vi "R4DataCollection.vi"(8 "error constant":errorcluster, 10 "Write Once":bool, 11 "LabVIEW Web Service":refnum<class "Web Service.lvclass">) -> (0 "error out":errorcluster={"status"=FALSE, "code"=0, "source"="0"})   [LabVIEW 2016]
uses:
  <vilib>/wsapi/Web Service.lvclass
  <vilib>/Platform/TimedLoop/XDataNode/timing_clust.ctl
  <vilib>/Platform/TimedLoop/XDataNode/nitl_modes.ctl
  <vilib>/Platform/TimedLoop/XDataNode/wakeup.ctl
  <vilib>/Platform/TimedLoop/XDataNode/XDataNode.xnode
  <vilib>/Platform/TimedLoop/XDataNode/XDNodeRunTimeDep.lvlib
  <vilib>/ptbypt/NI_PtbyPt.lvlib
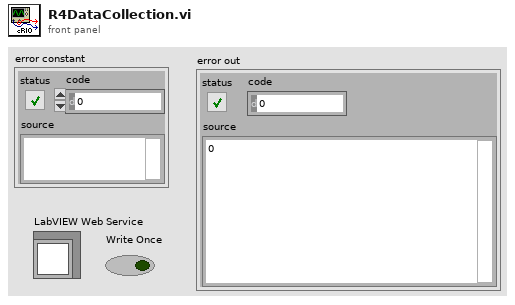
[diagram p1: front panel]
types:
  T1 = typedef "XDNodeRunTimeDep.lvlib/timing_clust.ctl" = cluster{"Expected End [f-1]":u64, "Actual End [f-1]":u64, "Finished Late? [f-1]":bool, "Expected End [i-1]":u64, "Actual End [i-1]":u64, "Finished Late? [i-1]":bool, "Expected Start [i]":u64, "Actual Start [i]":u64, "Expected Start [f]":u64, "Actual Start [f]":u64, "Source Name":string, "Structure Name":string, "Period":i64, "Deadline":i64, "Offset":i64, "Start":i64, "Priority":i32, "Timeout":i32, "Mode":T2, "Wakeup Reason":T3, "Error":errorcluster, "Source Type":string, "Secondary Source Type":string, "Global End Time":u64, "Global Start Time":u64, "Frame Duration":u64, "Iteration Duration":u64, "Assigned CPU":i32, "I/O Scan Engine Mode":u32}
  T2 = typedef "XDNodeRunTimeDep.lvlib/nitl_modes.ctl" = enum32{"No Change", "Process missed periods, maintain original phase", "Discard missed periods, maintain original phase", "Process missed periods, ignore original phase", "Discard missed periods, ignore original phase"}
  T3 = typedef "XDNodeRunTimeDep.lvlib/wakeup.ctl" = enum32{"Normal", "Aborted", "Asynchronous wakeup", "Timing source error", "Timed loop error", "Timeout"}
  T4 = cluster{"Media Pump":bool, "Water Pump":bool, "Gas Pump":bool, "Effluent Pump":bool, "Release Pump":bool}
  T5 = cluster{"Array of Double[0]":dbl, "Array of Double[1]":dbl, "Array of Double[2]":dbl, "Array of Double[3]":dbl, "Array of Double[4]":dbl, "Array of Double[5]":dbl, "Array of Double[6]":dbl, "Array of Double[7]":dbl, "Array of Double[8]":dbl}
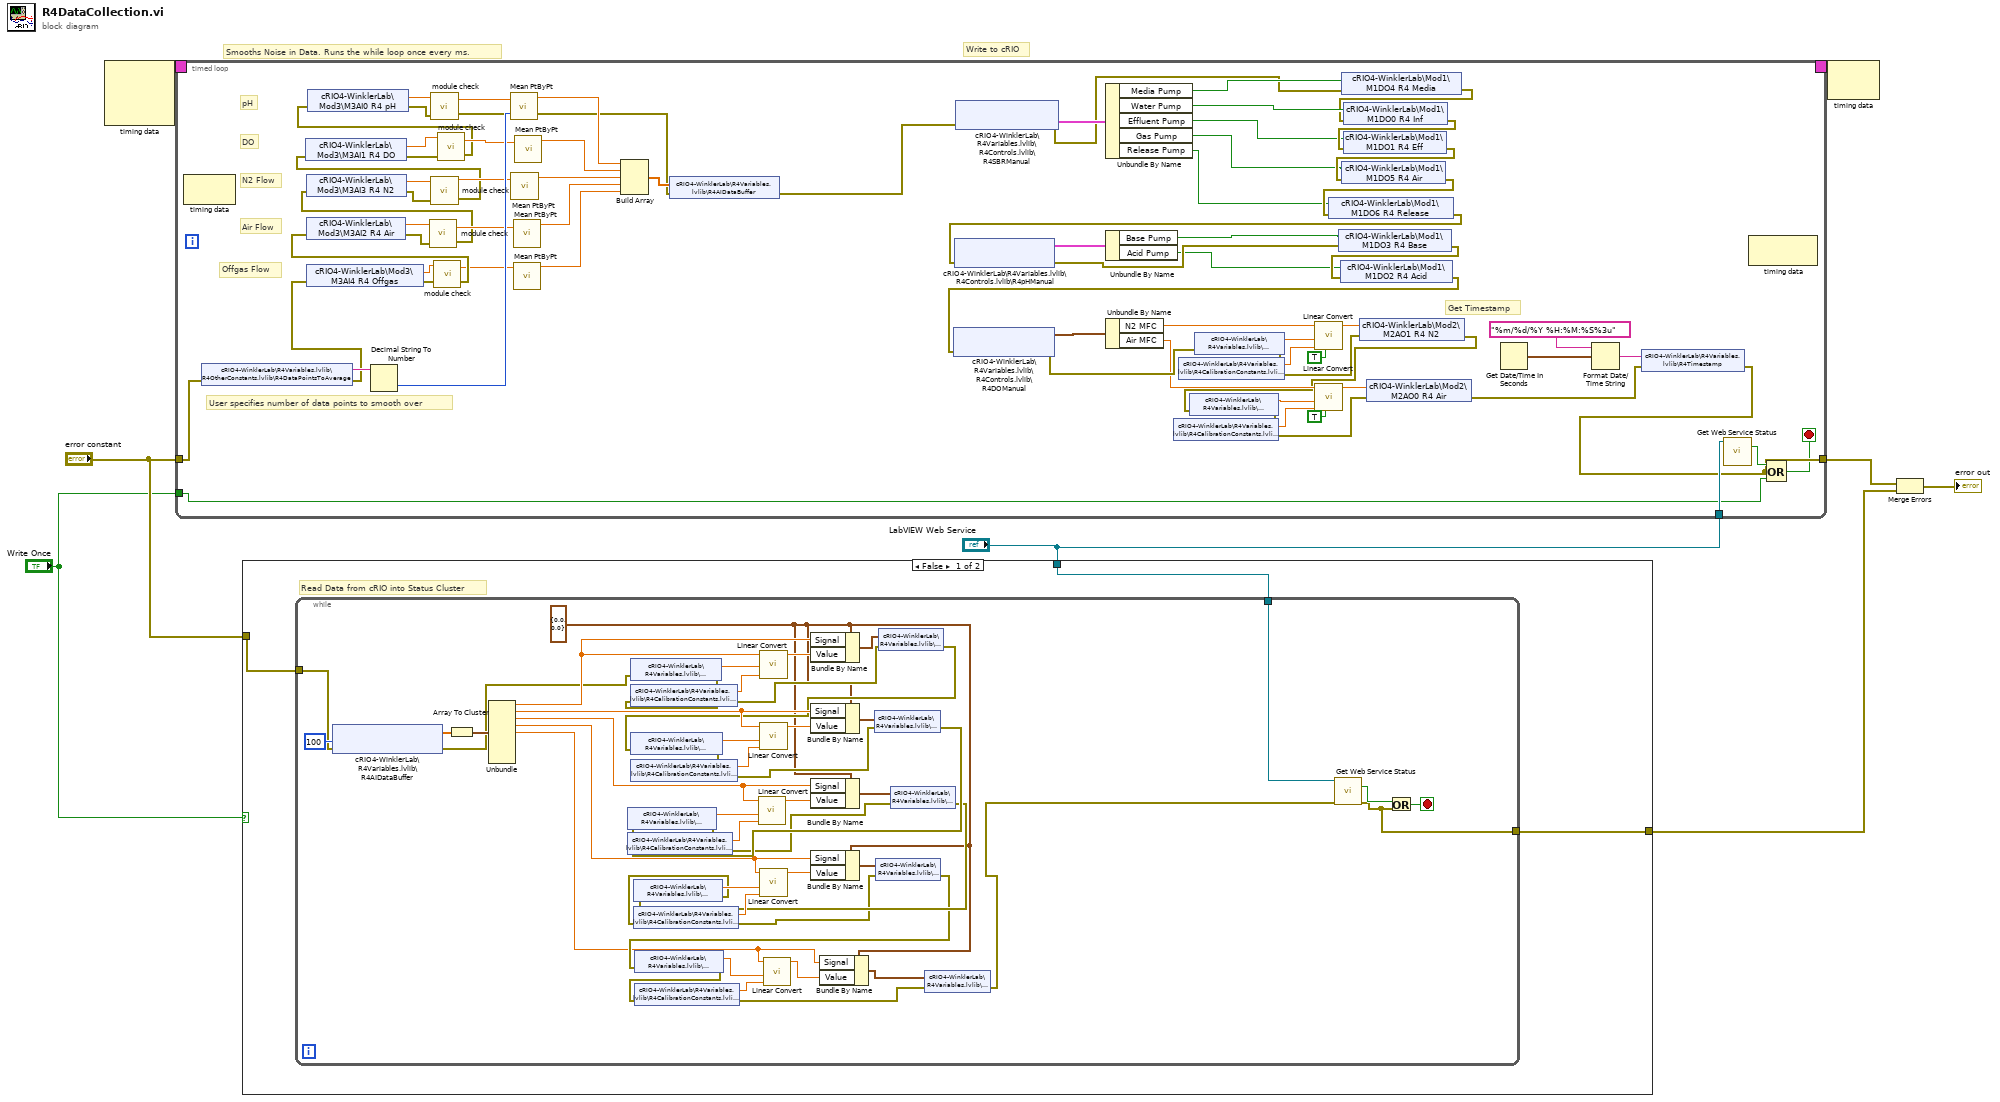
[diagram p0: block diagram]
diagram:
  # "Write to cRIO"
  # "Smooths Noise in Data. Runs the while loop once every ms."
  n1 = node-c288() -> (w8:T1)  [unwired: 3 in]
  n2 = timed-loop {
    timing: w8 -> [_]
    timing-out: [_] -> w7
    tunnel: "error constant" -> [w76]
    tunnel: "LabVIEW Web Service" -> [w72]
    tunnel: "Write Once" -> [w70]
    tunnel: [w69] -> w3
    stop <- w68 stop-if-true
    # "Offgas Flow"
    # "Get Timestamp"
    # "User specifies number of data points to smooth over"
    # "Air Flow"
    # "N2 Flow"
    # "DO"
    # "pH"
    n3 = node-c288() -> ()  [unwired: 1 in, 1 out]
    n4 = shared-variable "cRIO4-WinklerLab\\R4Variables.lvlib\\R4OtherConstants.lvlib\\R4DataPointsToAverage"(error in=w76) -> (w79:string, error out=w18:errorcluster)
    n5 = shared-variable "cRIO4-WinklerLab\\Mod3\\M3AI4 R4 Offgas"(error in=w18) -> (w20:dbl, error out=w19:errorcluster)
    n6 = Decimal String To Number(string=w79) -> (number=w67:i32)  [unwired: 2 in, 1 out]
    n7 = call "module check.vi"("error in"=w19, "Value"=w20) -> ("error constant"=w17:errorcluster, "Value out"=w16:dbl)  [unwired: 1 in]
    n8 = shared-variable "cRIO4-WinklerLab\\Mod3\\M3AI2 R4 Air"(error in=w17) -> (w43:dbl, error out=w44:errorcluster)
    n9 = call "module check.vi"("error in"=w44, "Value"=w43) -> ("error constant"=w40:errorcluster, "Value out"=w45:dbl)  [unwired: 1 in]
    n10 = shared-variable "cRIO4-WinklerLab\\Mod3\\M3AI3 R4 N2"(error in=w40) -> (w41:dbl, error out=w42:errorcluster)
    n11 = call "module check.vi"("error in"=w42, "Value"=w41) -> ("error constant"=w37:errorcluster, "Value out"=w46:dbl)  [unwired: 1 in]
    n12 = shared-variable "cRIO4-WinklerLab\\Mod3\\M3AI1 R4 DO"(error in=w37) -> (w38:dbl, error out=w39:errorcluster)
    n13 = call "module check.vi"("error in"=w39, "Value"=w38) -> ("error constant"=w34:errorcluster, "Value out"=w47:dbl)  [unwired: 1 in]
    n14 = shared-variable "cRIO4-WinklerLab\\Mod3\\M3AI0 R4 pH"(error in=w34) -> (w36:dbl, error out=w35:errorcluster)
    n15 = call "module check.vi"("error in"=w35, "Value"=w36) -> ("error constant"=w48:errorcluster, "Value out"=w49:dbl)  [unwired: 1 in]
    n16 = call <vilib>:"Mean PtByPt.vi"("x"=w49, "sample length"=w67) -> ("mean"=w66:dbl)  [unwired: 2 in, 1 out]
    n17 = call <vilib>:"Mean PtByPt.vi"("x"=w46) -> ("mean"=w64:dbl)  [unwired: 3 in, 1 out]
    n18 = call <vilib>:"Mean PtByPt.vi"("x"=w45) -> ("mean"=w65:dbl)  [unwired: 3 in, 1 out]
    n19 = call <vilib>:"Mean PtByPt.vi"("x"=w16) -> ("mean"=w15:dbl)  [unwired: 3 in, 1 out]
    n20 = call <vilib>:"Mean PtByPt.vi"("x"=w47) -> ("mean"=w63:dbl)  [unwired: 3 in, 1 out]
    n21 = Build Array(w66, w63, w64, w65, w15) -> (w83:dbl[])
    n22 = shared-variable "cRIO4-WinklerLab\\R4Variables.lvlib\\R4AIDataBuffer"(w83, error in=w48) -> (error out=w75:errorcluster)
    n23 = shared-variable "cRIO4-WinklerLab\\R4Variables.lvlib\\R4Controls.lvlib\\R4SBRManual"(error in=w75) -> (w78:T4, error out=w10:errorcluster)  [unwired: 1 in, 1 out]
    n24 = Unbundle By Name(w78) -> ("Media Pump"=w11:bool, "Water Pump"=w28:bool, "Effluent Pump"=w27:bool, "Gas Pump"=w26:bool, "Release Pump"=w25:bool)
    n25 = shared-variable "cRIO4-WinklerLab\\Mod1\\M1DO4 R4 Media"(w11, error in=w10) -> (error out=w9:errorcluster)
    n26 = shared-variable "cRIO4-WinklerLab\\Mod1\\M1DO0 R4 Inf"(w28, error in=w9) -> (error out=w33:errorcluster)
    n27 = shared-variable "cRIO4-WinklerLab\\Mod1\\M1DO1 R4 Eff"(w27, error in=w33) -> (error out=w32:errorcluster)
    n28 = shared-variable "cRIO4-WinklerLab\\Mod1\\M1DO5 R4 Air"(w26, error in=w32) -> (error out=w31:errorcluster)
    n29 = shared-variable "cRIO4-WinklerLab\\Mod1\\M1DO6 R4 Release"(w25, error in=w31) -> (error out=w24:errorcluster)
    n30 = shared-variable "cRIO4-WinklerLab\\R4Variables.lvlib\\R4Controls.lvlib\\R4pHManual"(error in=w24) -> (w77:cluster{"Acid Pump":bool, "Base Pump":bool}, error out=w23:errorcluster)  [unwired: 1 in, 1 out]
    n31 = Unbundle By Name(w77) -> ("Base Pump"=w22:bool, "Acid Pump"=w21:bool)
    n32 = shared-variable "cRIO4-WinklerLab\\Mod1\\M1DO3 R4 Base"(w22, error in=w23) -> (error out=w30:errorcluster)
    n33 = shared-variable "cRIO4-WinklerLab\\Mod1\\M1DO2 R4 Acid"(w21, error in=w30) -> (error out=w29:errorcluster)
    n34 = shared-variable "cRIO4-WinklerLab\\R4Variables.lvlib\\R4Controls.lvlib\\R4DOManual"(error in=w29) -> (w74:cluster{"Air MFC":dbl, "N2 MFC":dbl}, error out=w73:errorcluster)  [unwired: 1 in, 1 out]
    n35 = Unbundle By Name(w74) -> ("N2 MFC"=w62:dbl, "Air MFC"=w61:dbl)
    n36 = shared-variable "cRIO4-WinklerLab\\R4Variables.lvlib\\R4CalibrationConstants.lvlib\\R4N2Slope"(error in=w73) -> (w56:dbl, error out=w54:errorcluster)
    n37 = shared-variable "cRIO4-WinklerLab\\R4Variables.lvlib\\R4CalibrationConstants.lvlib\\R4N2Intercept"(error in=w54) -> (w55:dbl, error out=w13:errorcluster)
    n38 = call "Linear Convert.vi"("Inverse?"=TRUE, "Intercept"=w55, "Slope"=w56, "Signal"=w62) -> ("Result"=w14:dbl)  [unwired: 7 in]
    n39 = shared-variable "cRIO4-WinklerLab\\Mod2\\M2AO1 R4 N2"(w14, error in=w13) -> (error out=w12:errorcluster)
    n40 = shared-variable "cRIO4-WinklerLab\\R4Variables.lvlib\\R4CalibrationConstants.lvlib\\R4AirSlope"(error in=w12) -> (w58:dbl, error out=w53:errorcluster)
    n41 = shared-variable "cRIO4-WinklerLab\\R4Variables.lvlib\\R4CalibrationConstants.lvlib\\R4AirIntercept"(error in=w53) -> (w57:dbl, error out=w51:errorcluster)
    n42 = call "Linear Convert.vi"("Inverse?"=TRUE, "Intercept"=w57, "Slope"=w58, "Signal"=w61) -> ("Result"=w50:dbl)  [unwired: 7 in]
    n43 = shared-variable "cRIO4-WinklerLab\\Mod2\\M2AO0 R4 Air"(w50, error in=w51) -> (error out=w52:errorcluster)
    n44 = Get Date/Time In Seconds() -> (seconds since 1Jan1904=w81:timestamp)
    n45 = Format Date/Time String(time format string (%c)="%m/%d/%Y %H:%M:%S%3u", seconds (now)=w81) -> (date/time string=w80:string)  [unwired: 1 in]
    n46 = shared-variable "cRIO4-WinklerLab\\R4Variables.lvlib\\R4Timestamp"(w80, error in=w52) -> (error out=w69:errorcluster)
    n47 = call <vilib>:"Get Web Service Status.vi"("LabVIEW Web Service"=w72) -> ("service stopping?"=w71:bool)  [unwired: 12 in, 2 out]
    n48 = node-c288() -> ()  [unwired: 1 in, 1 out]
    n49 = Compound Arithmetic op=OR(w71, w69, w70) -> (w68:bool)
  }
  n50 = case shown="False" "Write Once" {
    tunnel: "error constant" -> [w88 w139]
    tunnel: "LabVIEW Web Service" -> [w87 _]
    tunnel: [w86 w139] -> w2
    frame False {
      # "Read Data from cRIO into Status Cluster"
      n51 = while {
        tunnel: w88 -> [w104]
        tunnel: [w103] -> w86
        tunnel: w87 -> [w102]
        stop <- w129 stop-if-true
        w89 = cluster{"Signal":dbl, "Value":dbl} {"Signal"=0.0, "Value"=0.0} ("Analog Input")
        n52 = shared-variable "cRIO4-WinklerLab\\R4Variables.lvlib\\R4AIDataBuffer"(error in=w104, u32 100 ("milliseconds to wait")) -> (w136:dbl[], error out=w114:errorcluster)  [unwired: 1 out]
        n53 = Array To Cluster(array=w136) -> (cluster=w138:T5)
        n54 = Unbundle(w138) -> ("Array of Double[0]"=w134:dbl, "Array of Double[1]"=w133:dbl, "Array of Double[2]"=w122:dbl, "Array of Double[3]"=w121:dbl, "Array of Double[4]"=w91:dbl)  [unwired: 4 out]
        n55 = shared-variable "cRIO4-WinklerLab\\R4Variables.lvlib\\R4CalibrationConstants.lvlib\\R4pHSlope"(error in=w114) -> (w127:dbl, error out=w113:errorcluster)
        n56 = shared-variable "cRIO4-WinklerLab\\R4Variables.lvlib\\R4CalibrationConstants.lvlib\\R4pHIntercept"(error in=w113) -> (w128:dbl, error out=w99:errorcluster)
        n57 = call "Linear Convert.vi"("Intercept"=w128, "Slope"=w127, "Signal"=w134) -> ("Result"=w135:dbl)  [unwired: 8 in]
        n58 = Bundle By Name(cluster=w89, "Signal"=w134, "Value"=w135) -> (w100:cluster{"Signal":dbl, "Value":dbl})
        n59 = shared-variable "cRIO4-WinklerLab\\R4Variables.lvlib\\R4Signals.lvlib\\R4pH"(w100, error in=w99) -> (error out=w101:errorcluster)
        n60 = shared-variable "cRIO4-WinklerLab\\R4Variables.lvlib\\R4CalibrationConstants.lvlib\\R4DOSlope"(error in=w101) -> (w126:dbl, error out=w112:errorcluster)
        n61 = shared-variable "cRIO4-WinklerLab\\R4Variables.lvlib\\R4CalibrationConstants.lvlib\\R4DOIntercept"(error in=w112) -> (w125:dbl, error out=w111:errorcluster)
        n62 = call "Linear Convert.vi"("Intercept"=w125, "Slope"=w126, "Signal"=w133) -> ("Result"=w131:dbl)  [unwired: 8 in]
        n63 = Bundle By Name(cluster=w89, "Signal"=w133, "Value"=w131) -> (w132:cluster{"Signal":dbl, "Value":dbl})
        n64 = shared-variable "cRIO4-WinklerLab\\R4Variables.lvlib\\R4Signals.lvlib\\R4DO"(w132, error in=w111) -> (error out=w110:errorcluster)
        n65 = shared-variable "cRIO4-WinklerLab\\R4Variables.lvlib\\R4CalibrationConstants.lvlib\\R4N2Slope"(error in=w110) -> (w118:dbl, error out=w109:errorcluster)
        n66 = shared-variable "cRIO4-WinklerLab\\R4Variables.lvlib\\R4CalibrationConstants.lvlib\\R4N2Intercept"(error in=w109) -> (w117:dbl, error out=w108:errorcluster)
        n67 = call "Linear Convert.vi"("Intercept"=w117, "Slope"=w118, "Signal"=w122) -> ("Result"=w123:dbl)  [unwired: 8 in]
        n68 = Bundle By Name(cluster=w89, "Signal"=w122, "Value"=w123) -> (w115:cluster{"Signal":dbl, "Value":dbl})
        n69 = shared-variable "cRIO4-WinklerLab\\R4Variables.lvlib\\R4Signals.lvlib\\R4N2"(w115, error in=w108) -> (error out=w107:errorcluster)
        n70 = shared-variable "cRIO4-WinklerLab\\R4Variables.lvlib\\R4CalibrationConstants.lvlib\\R4AirSlope"(error in=w107) -> (w120:dbl, error out=w106:errorcluster)
        n71 = shared-variable "cRIO4-WinklerLab\\R4Variables.lvlib\\R4CalibrationConstants.lvlib\\R4AirIntercept"(error in=w106) -> (w119:dbl, error out=w105:errorcluster)
        n72 = call "Linear Convert.vi"("Intercept"=w119, "Slope"=w120, "Signal"=w121) -> ("Result"=w124:dbl)  [unwired: 8 in]
        n73 = Bundle By Name(cluster=w89, "Signal"=w121, "Value"=w124) -> (w116:cluster{"Signal":dbl, "Value":dbl})
        n74 = shared-variable "cRIO4-WinklerLab\\R4Variables.lvlib\\R4Signals.lvlib\\R4Air"(w116, error in=w105) -> (error out=w95:errorcluster)
        n75 = shared-variable "cRIO4-WinklerLab\\R4Variables.lvlib\\R4CalibrationConstants.lvlib\\R4AirSlope"(error in=w95) -> (w98:dbl, error out=w90:errorcluster)
        n76 = shared-variable "cRIO4-WinklerLab\\R4Variables.lvlib\\R4CalibrationConstants.lvlib\\R4AirIntercept"(error in=w90) -> (w97:dbl, error out=w96:errorcluster)
        n77 = call "Linear Convert.vi"("Intercept"=w97, "Slope"=w98, "Signal"=w91) -> ("Result"=w92:dbl)  [unwired: 8 in]
        n78 = Bundle By Name(cluster=w89, "Signal"=w91, "Value"=w92) -> (w93:cluster{"Signal":dbl, "Value":dbl})
        n79 = shared-variable "cRIO4-WinklerLab\\R4Variables.lvlib\\R4Signals.lvlib\\R4Off"(w93, error in=w96) -> (error out=w94:errorcluster)
        n80 = call <vilib>:"Get Web Service Status.vi"("LabVIEW Web Service"=w102, "error in (no error)"=w94) -> ("service stopping?"=w130:bool, "error out"=w103:errorcluster)  [unwired: 11 in, 1 out]
        n81 = Or(x=w130, y=w103) -> (x .or. y?=w129:bool)
      }
    }
    frame True {
    }
  }
  n82 = node-c288(w7) -> ()  [unwired: 1 out]
  n83 = Merge Errors(w3, w2) -> (→"error out":errorcluster)
